vi "weufgiqwef.vi"() -> ()   [LabVIEW 2020]
panel:
  in  "Switch":bool
  out "LED":bool
  in  "stop":bool
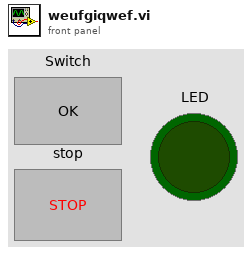
[diagram p1: front panel]
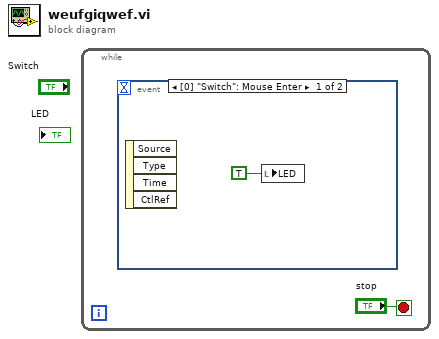
[diagram p0: block diagram]
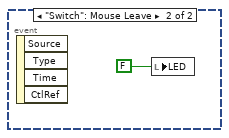
[diagram p2: hidden frame]
diagram:
  n1 = while {
    stop <- "stop" stop-if-true
    n2 = event shown="[0] \"Switch\": Mouse Enter" {
      selector: _ -> [_ _]
      dyn-events: _ -> [_ _]
      timeout: _ -> [_ _]
      event "Switch": Mouse Enter {
        n3 = event-data() -> ()  [unwired: 1 in, 4 out]
        n4 = local write "LED"(TRUE ("Boolean")) -> ()
      }
      event "Switch": Mouse Leave {
        n5 = event-data() -> ()  [unwired: 1 in, 4 out]
        n6 = local write "LED"(FALSE ("Boolean")) -> ()
      }
    }
  }
